vi "hse-application_ApplicationShutdown.vi"(8 "error in":errorcluster) -> (0 "error out":errorcluster)   [LabVIEW 2014, in "hse-application.lvclass"]
doc: "Stops and frees all hse resources.\n\n\n\n____\nHAMPEL SOFTWARE ENGINEERING v0.12.0 (2018-09-13 18:21)"
uses:
  hse-application.lvclass
  hse-misc/Error/Error_Labels.ctl
  hse-misc/Error/Error_Helper_RaiseErrorFromLabel.vi
  hse-misc/hse-misc.lvlib
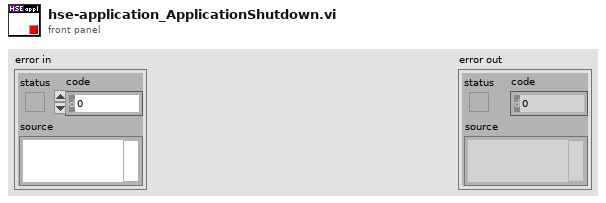
[diagram p1: front panel]
types:
  T1 = typedef "hse-misc.lvlib/Error_Labels.ctl" = enum16{"=== GENERIC ===", "Unexpected / unknown error", "Timeout", "Device or resource not found", "Expected (handled) error", "Module or VI not executable", "Server shutting down", "File not found", "Cancelled by user", "Invalid parameter", "Configuration type invalid", "Configuration token not found", "Error occurred parsing configuration string", "External program returned with error", "Unexpected data", "Unknown message", "Attribute not found (in a variant or tree)", "Number of elements mismatch (e.g. in an array)", "Maximum number of attempts (e.g. for a reconnection)", "Input out of range", "Registry file not found or not readable", "Registry type mismatch", "Project name mismatch", "System identifier mismatch", "Configuration file not found", "Checking remote path failed", "Establishing data connection failed", "The network operation exceeded the time limit", "Network is down/unreachable/reset", "The specified port or network address is currently in use", "=== NI DISCOVERY PROTOCOL ===", "=== APPLICATION BUILDER ===", "=== GIT ===", "Return code != 0", "=== FGPA ===", "Generic FPGA error", "Timeout general", "Timeout FIFO", "Timeout DMA", "Timeout Handshake", "Loop time exceeded", "=== IO ===", "=== PROFINET ===", "=== USER INTERFACE ===", "=== GENERIC NETWORKING (NET-TX & NET-RX ==="}
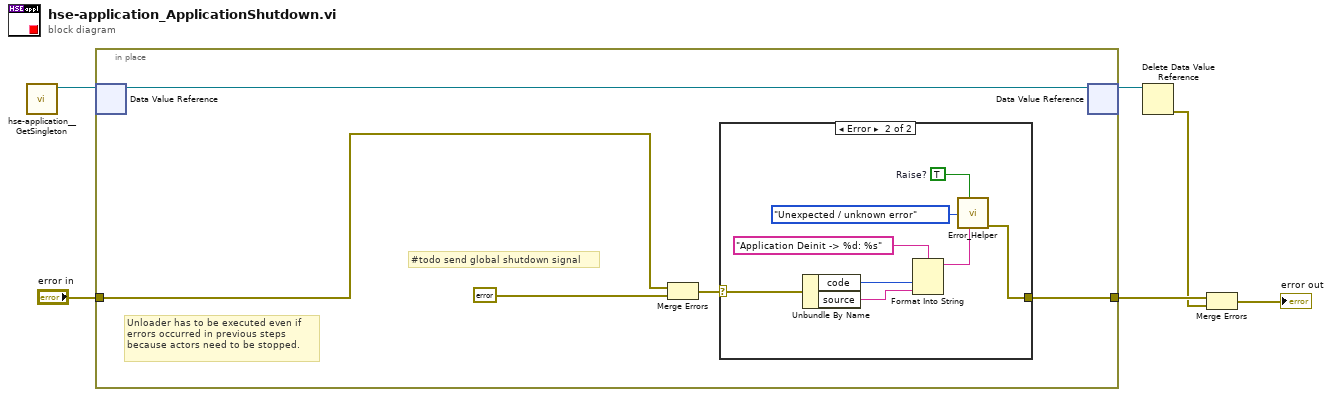
[diagram p0: block diagram]
diagram:
  n1 = call "hse-application__GetSingleton.vi"() -> ("ApplicationClass DVR"=w5:refnum<data-value>)  [unwired: 10 in, 1 out]
  n2 = in-place {
    in-place-border: "error in" -> [w9]
    in-place-border: [w7] -> w3
    # "#todo send global shutdown signal"
    # "Unloader has to be executed even if \nerrors occurred in previous steps \nbecause actors need to be stopped."
    n3 = in-place-dvr #1(w5) -> (w8:refnum<class "hse-application.lvclass">)  [unwired: 1 out]
    n4 = Merge Errors(w9, errorcluster {"status"=FALSE, "code"=0, "source"=""} ("Error In")) -> (w10:errorcluster)
    n5 = case shown="Error" w10 {
      selector: w10 -> [w12 w16]
      tunnel: [w12 w15] -> w7
      frame No Error {
      }
      frame Error {
        w14 = TRUE  # Raise?
        n6 = Unbundle By Name(w16) -> ("code"=w20:i32, "source"=w19:string)
        n7 = Format Into String(format string="Application Deinit -> %d: %s", w20, w19) -> (resulting string=w17:string)  [unwired: 2 in, 1 out]
        n8 = call-poly "Error_Helper.vi"("Additional Info"=w17, "Raise?"=w14, "Error Labels"=Error_Labels."Unexpected / unknown error") -> ("Error Out"=w15:errorcluster)  [unwired: 8 in]
      }
    }
    n9 = in-place-dvr #1(w8) -> (w4:refnum<data-value>)  [unwired: 1 out]
  }
  n10 = Delete Data Value Reference(data value reference=w4) -> (error out=w2:errorcluster)  [unwired: 1 in, 1 out]
  n11 = Merge Errors(w3, w2) -> (→"error out":errorcluster)
